vi "Check For Messages.vi"(9 "Term Char":string="\r\n", 11 "Input String":string) -> (0 "found?":bool, 1 "data":u8[](array[numeric]), 3 "Remaining String":string)   [LabVIEW 2012, in "ASCII Data Unit.lvclass"]
uses:
  ASCII Data Unit.lvclass
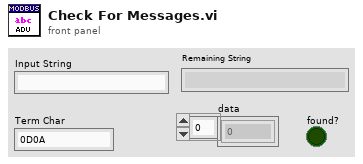
[diagram p1: front panel]
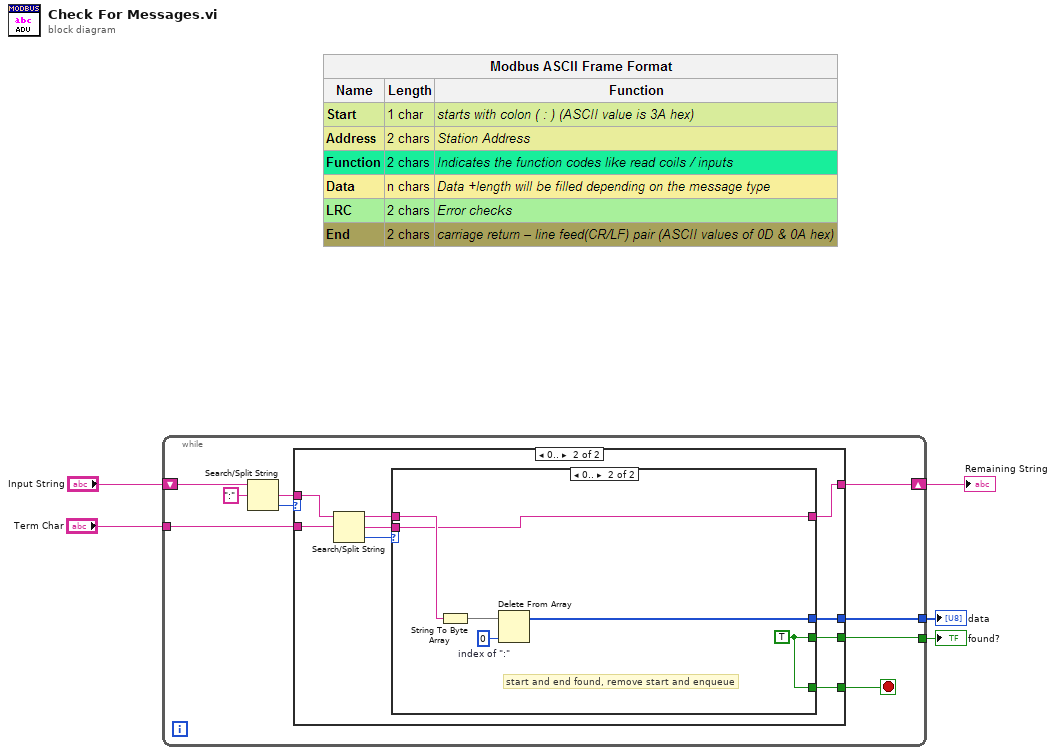
[diagram p0: block diagram]
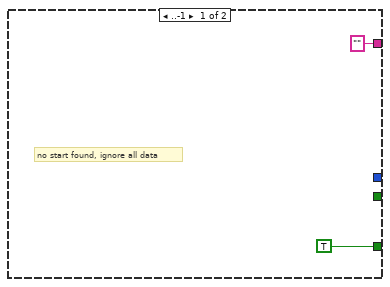
[diagram p2: hidden frame]
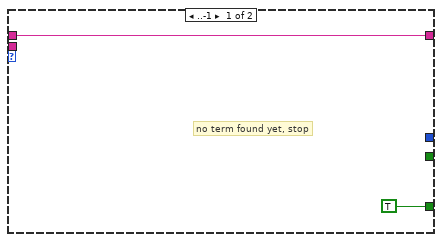
[diagram p3: hidden frame]
diagram:
  n1 = while {
    tunnel: "Term Char" -> [w12]
    shift-right: [w9] -> w3
    shift-left: "Input String" -> [w14]
    tunnel: [w7] -> w2
    tunnel: [w6] -> w1
    stop <- w8 stop-if-true
    n2 = Search/Split String(string=w14, search string/char (-)=":") -> (match + rest of string=w11:string, offset of match=w10:i32)  [unwired: 1 in, 1 out]
    n3 = case shown="0.." w10 {
      tunnel: w12 -> [_ w25]
      tunnel: w11 -> [_ w24]
      tunnel: ["" ("Input String") w21] -> w9
      tunnel: [TRUE w22] -> w8
      tunnel: [_ w18] -> w7
      tunnel: [_ w17] -> w6
      frame ..-1 {
        # "no start found, ignore all data"
      }
      frame 0.. {
        n4 = Search/Split String(string=w24, search string/char (-)=w25) -> (substring before match=w20:string, match + rest of string=w19:string, offset of match=w23:i32)  [unwired: 1 in]
        n5 = case shown="0.." w23 {
          tunnel: [TRUE w28] -> w22
          tunnel: [w26 w30] -> w21
          tunnel: w20 -> [w26 w33]
          tunnel: w19 -> [_ w30]
          tunnel: [_ w29] -> w18
          tunnel: [_ w28] -> w17
          frame ..-1 {
            # "no term found yet, stop"
          }
          frame 0.. {
            w28 = TRUE
            w31 = 0  # index of ":"
            # "start and end found, remove start and enqueue"
            n6 = String To Byte Array(string=w33) -> (unsigned byte array=w32:u8[])
            n7 = Delete From Array(array=w32, index=w31) -> (array with subset deleted=w29:u8[])  [unwired: 1 in, 1 out]
          }
        }
      }
    }
  }
  "Remaining String" <- w3
  "data" <- w2
  "found?" <- w1
